vi "2021_01_Init.vi"(8 "Error In":errorcluster, 11 "Object in":refnum<class "2021_01.lvclass">) -> (0 "Error Out":errorcluster, 3 "object out":refnum<class "2021_01.lvclass">)   [LabVIEW 2020]
uses:
  2021_01.lvclass/2021_01.ctl
  2021_01.lvclass
  C:/Projects/AdventCode/PuzzleBase_class/PuzzleBase.lvclass
  C:/Projects/AdventCode/PuzzleClasses/2021_01_class/2021_01.lvclass
  PuzzleBase_class/PuzzleBase.lvclass
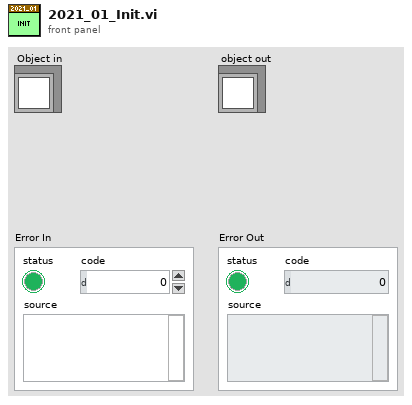
[diagram p1: front panel]
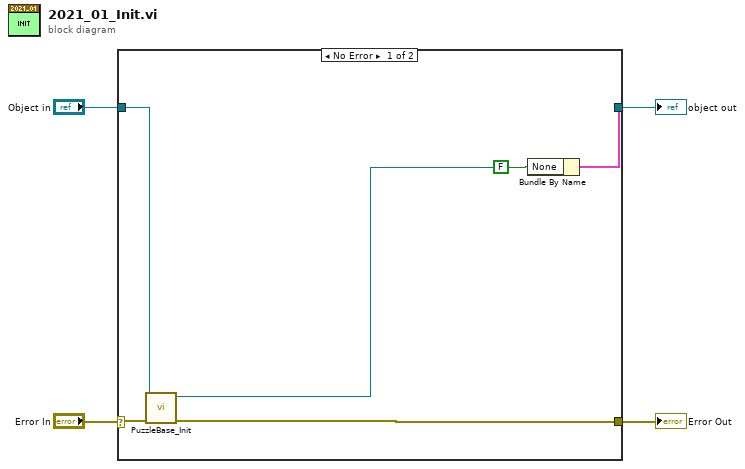
[diagram p0: block diagram]
diagram:
  n1 = case shown="No Error" "Error In" {
    selector: "Error In" -> [w8 w11]
    tunnel: [w10 w12] -> w4
    tunnel: "Object in" -> [w6 w12]
    tunnel: [w7 w11] -> w1
    frame No Error {
      n2 = call "PuzzleBase_Init.vi"("Error In"=w8, "object in"=w6) -> ("Error Out"=w7:errorcluster, "object out"=w5:refnum<class "PuzzleBase.lvclass">)  [unwired: 8 in]
      n3 = Bundle By Name(cluster=w5, "None"=FALSE) -> (w10:cluster{})
    }
    frame Error {
    }
  }
  "object out" <- w4
  "Error Out" <- w1
